vi "King in Danger.vi"(0 "King Index":i32=2, 1 "Opp. King Index":i32=6, 5 "Count":i32[](array[numeric])=[1, 0, 0, 2, 0, 2, 0, 0, 0, 0, 1, 1, 0, 1, 0, 0, 0, 0, 0, 0, 0, 0, 0, 0, 0, 0, 0, 0, 1, 0, 0, 0, 0, 1, 0, 1, 1, 0, 1, 1, 0, 1, 0, 1, 0, 0, 2, 1, 0], 7 "Opp Team Cells":i32[](array[numeric])=[0, 5, 13, 28, 35, 36, 39, 41, 43], 9 "1D Board":T1[](array[typedef])=[{"Team"=1, "Occu."=enum."C", "Count"=1}, {"Team"=0, "Occu."=enum."N", "Count"=0}, {"Team"=2, "Occu."=enum."K", "Count"=0}, {"Team"=2, "Occu."=enum."C", "Count"=2}, {"Team"=0, "Occu."=enum."N", "Count"=0}, {"Team"=1, "Occu."=enum."C", "Count"=2}, {"Team"=1, "Occu."=enum."K", "Count"=0}, {"Team"=0, "Occu."=enum."N", "Count"=0}, {"Team"=0, "Occu."=enum."N", "Count"=0}, {"Team"=0, "Occu."=enum."N", "Count"=0}, {"Team"=2, "Occu."=enum."C", "Count"=1}, {"Team"=2, "Occu."=enum."C", "Count"=1}, {"Team"=0, "Occu."=enum."N", "Count"=0}, {"Team"=1, "Occu."=enum."C", "Count"=1}, {"Team"=0, "Occu."=enum."N", "Count"=0}, {"Team"=0, "Occu."=enum."N", "Count"=0}, {"Team"=0, "Occu."=enum."N", "Count"=0}, {"Team"=0, "Occu."=enum."N", "Count"=0}, {"Team"=0, "Occu."=enum."N", "Count"=0}, {"Team"=0, "Occu."=enum."N", "Count"=0}, {"Team"=0, "Occu."=enum."N", "Count"=0}, {"Team"=0, "Occu."=enum."N", "Count"=0}, {"Team"=0, "Occu."=enum."N", "Count"=0}, {"Team"=0, "Occu."=enum."N", "Count"=0}, {"Team"=0, "Occu."=enum."N", "Count"=0}, {"Team"=0, "Occu."=enum."N", "Count"=0}, {"Team"=0, "Occu."=enum."N", "Count"=0}, {"Team"=0, "Occu."=enum."N", "Count"=0}, {"Team"=1, "Occu."=enum."C", "Count"=1}, {"Team"=0, "Occu."=enum."N", "Count"=0}, {"Team"=0, "Occu."=enum."N", "Count"=0}, {"Team"=0, "Occu."=enum."N", "Count"=0}, {"Team"=0, "Occu."=enum."N", "Count"=0}, {"Team"=2, "Occu."=enum."C", "Count"=1}, {"Team"=0, "Occu."=enum."N", "Count"=0}, {"Team"=1, "Occu."=enum."C", "Count"=1}, {"Team"=1, "Occu."=enum."C", "Count"=1}, {"Team"=0, "Occu."=enum."N", "Count"=0}, {"Team"=2, "Occu."=enum."C", "Count"=1}, {"Team"=1, "Occu."=enum."C", "Count"=1}, {"Team"=0, "Occu."=enum."N", "Count"=0}, {"Team"=1, "Occu."=enum."C", "Count"=1}, {"Team"=0, "Occu."=enum."N", "Count"=0}, {"Team"=1, "Occu."=enum."C", "Count"=1}, {"Team"=0, "Occu."=enum."N", "Count"=0}, {"Team"=0, "Occu."=enum."N", "Count"=0}, {"Team"=2, "Occu."=enum."C", "Count"=2}, {"Team"=2, "Occu."=enum."C", "Count"=1}, {"Team"=0, "Occu."=enum."N", "Count"=0}], 11 "error in (no error)":errorcluster, 12 "Team":i32=1) -> (4 "King in Danger?":bool, 6 "Cell Index":i32, 8 "Swap to Kill?":bool, 15 "error out":errorcluster)   [LabVIEW 2014, in "Dragon Tamers.lvlib"]
uses:
  Dragon Tamers.lvlib
  Typedefs/Board Cell.ctl
  Typedefs/Cell Occupancy.ctl
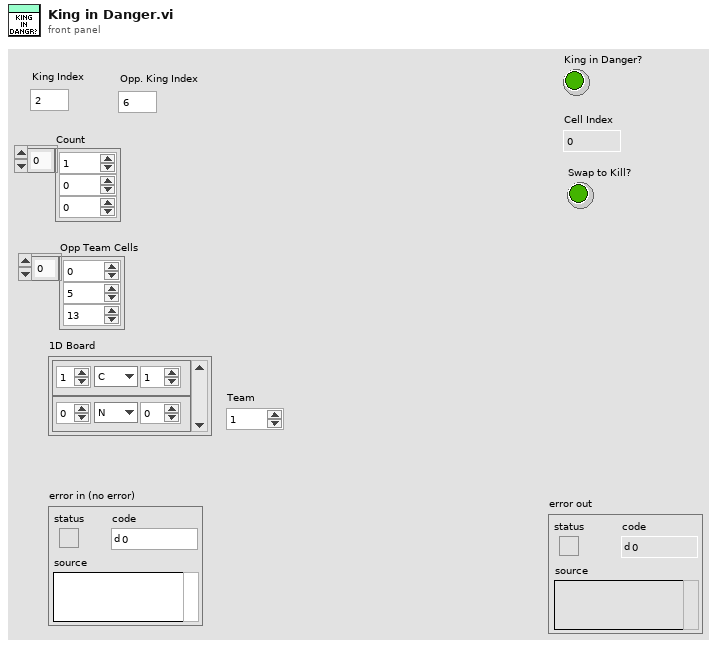
[diagram p1: front panel]
types:
  T1 = typedef "Dragon Tamers.lvlib/Board Cell.ctl" = cluster{"Team":i32, "Occu.":T2, "Count":i32}
  T2 = typedef "Dragon Tamers.lvlib/Cell Occupancy.ctl" = enum16{"N", "C", "K"}
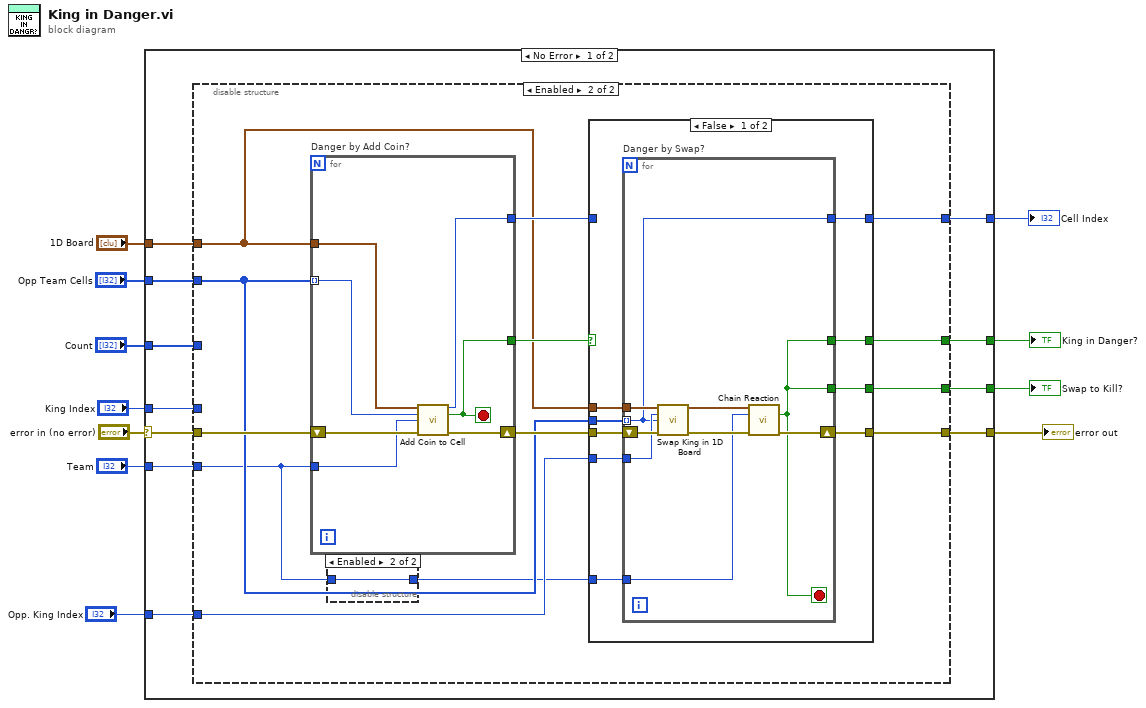
[diagram p0: block diagram]
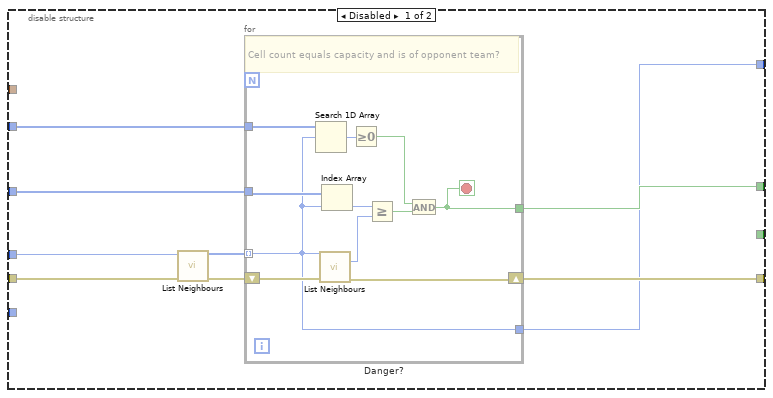
[diagram p2: hidden frame]
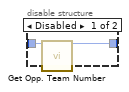
[diagram p3: hidden frame]
diagram:
  n1 = case shown="No Error" "error in (no error)" {
    selector: "error in (no error)" -> [w22 w87]
    tunnel: [w21 w87] -> w10
    tunnel: "King Index" -> [w20 _]
    tunnel: "Count" -> [w19 _]
    tunnel: [w18 _] -> w7
    tunnel: [w17 _] -> w6
    tunnel: "Opp Team Cells" -> [w16 _]
    tunnel: "1D Board" -> [w15 _]
    tunnel: "Team" -> [w14 _]
    tunnel: "Opp. King Index" -> [w13 _]
    tunnel: [w12 _] -> w1
    frame No Error {
      n2 = disable-structure shown="Enabled" {
        disable-tunnel: w22 -> [w29 w55]
        disable-tunnel: [w28 w53] -> w21
        disable-tunnel: w20 -> [w27 _]
        disable-tunnel: w19 -> [w26 _]
        disable-tunnel: [w25 w47] -> w18
        disable-tunnel: [w24 w45] -> w17
        disable-tunnel: w16 -> [w23 w52]
        disable-tunnel: w15 -> [_ w43]
        disable-tunnel: w14 -> [_ w50]
        disable-tunnel: w13 -> [_ w51]
        disable-tunnel: [_ w44] -> w12
        frame Disabled {
          n3 = call "List Neighbours.vi"("Cell Index"=w27, "error in (no error)"=w29) -> ("Neighbours"=w31:i32[], "error out"=w30:errorcluster)  [unwired: 11 in, 1 out]
          n4 = for "Danger?" {
            tunnel: w31 -> [w36] mode=indexing
            shift-right: [w39] -> w28
            shift-left: w30 -> [w42]
            tunnel: w26 -> [w41]
            tunnel: [w32] -> w25
            tunnel: [w36] -> w24
            tunnel: w23 -> [w37]
            stop <- w32 stop-if-true
            # "Cell count equals capacity and is of opponent team?"
            n5 = Search 1D Array(1D array=w37, element=w36) -> (index of element=w35:i32)  [unwired: 1 in]
            n6 = call "List Neighbours.vi"("Cell Index"=w36, "error in (no error)"=w42) -> ("Max Capacity"=w40:i32, "error out"=w39:errorcluster)  [unwired: 11 in, 1 out]
            n7 = Index Array(array=w41, index=w36) -> (element=w38:i32)
            n8 = Greater Or Equal To 0?(x=w35) -> (x >= 0?=w34:bool)
            n9 = Greater Or Equal?(x=w38, y=w40) -> (x >= y?=w33:bool)
            n10 = And(x=w34, y=w33) -> (x .and. y?=w32:bool)
          }
        }
        frame Enabled {
          n11 = for "Danger by Add Coin?" {
            tunnel: w43 -> [w85]
            tunnel: w50 -> [w84]
            tunnel: w52 -> [w83] mode=indexing
            tunnel: [w81] -> w48
            shift-right: [w82] -> w54
            shift-left: w55 -> [w86]
            tunnel: [w80] -> w46
            stop <- w81 stop-if-true
            n12 = call "Add Coin to Cell.vi"("1D Board Array"=w85, "Cell Index"=w83, "Team Number"=w84, "error in (no error)"=w86) -> ("Cell Index"=w80:i32, "Win?"=w81:bool, "error out"=w82:errorcluster)  [unwired: 7 in, 2 out]
          }
          n13 = disable-structure shown="Enabled" {
            disable-tunnel: w50 -> [w57 w58]
            disable-tunnel: [w56 w58] -> w49
            frame Disabled {
              n14 = call "Get Opp. Team Number.vi"("DT Team"=w57) -> ("Opp Team"=w56:i32)  [unwired: 14 in]
            }
            frame Enabled {
            }
          }
          n15 = case shown="False" w48 {
            selector: w48 -> [_ w79]
            tunnel: w54 -> [w67 w77]
            tunnel: [w66 w77] -> w53
            tunnel: w52 -> [w65 _]
            tunnel: w43 -> [w64 _]
            tunnel: w51 -> [w63 _]
            tunnel: w49 -> [w62 _]
            tunnel: [w61 w79] -> w47
            tunnel: w46 -> [_ w78]
            tunnel: [w60 w78] -> w45
            tunnel: [w59 _] -> w44
            frame False {
              n16 = for "Danger by Swap?" {
                shift-right: [w72] -> w66
                shift-left: w67 -> [w76]
                tunnel: w65 -> [w70] mode=indexing
                tunnel: w64 -> [w75]
                tunnel: w63 -> [w74]
                tunnel: w62 -> [w71]
                tunnel: [w69] -> w61
                tunnel: [w70] -> w60
                tunnel: [w69] -> w59
                stop <- w69 stop-if-true
                n17 = call "Swap King in 1D Board.vi"("1D Board"=w75, "King Index"=w74, "Cell Index"=w70, "error in (no error)"=w76) -> ("1D Board Out"=w68:T1[], "error out"=w73:errorcluster)  [unwired: 10 in]
                n18 = call "Chain Reaction.vi"("1D Board"=w68, "Team Number"=w71, "error in (no error)"=w73) -> ("Won?"=w69:bool, "error out"=w72:errorcluster)  [unwired: 9 in, 2 out]
              }
            }
            frame True {
            }
          }
        }
      }
    }
    frame Error {
    }
  }
  "error out" <- w10
  "King in Danger?" <- w7
  "Cell Index" <- w6
  "Swap to Kill?" <- w1
